vi "MH_WritePTURecordArr.vi"(0 "refnum":refnum<file>, 2 "TTTR Records":u32[](array[numeric]), 3 "error in":errorcluster) -> (6 "refnum en sortie":refnum<file>, 10 "error out":errorcluster)   [LabVIEW 2019]
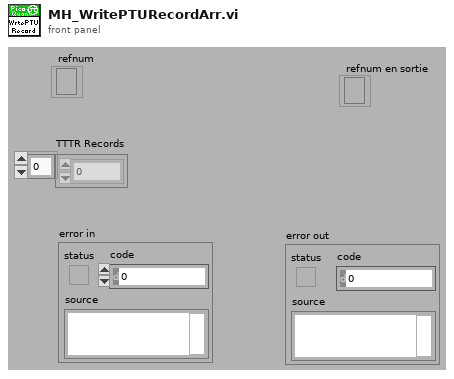
[diagram p1: front panel]
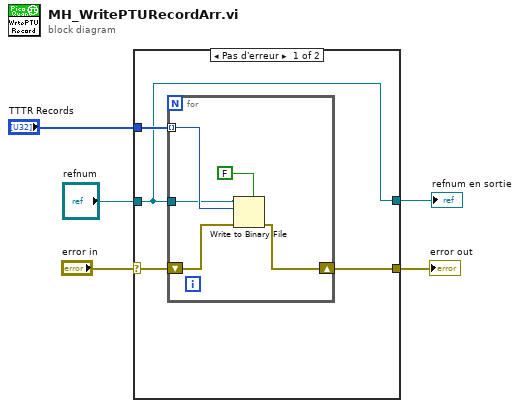
[diagram p0: block diagram]
diagram:
  n1 = case shown="Pas d'erreur" "error in" {
    selector: "error in" -> [w8 w16]
    tunnel: "refnum" -> [w6 w15]
    tunnel: [w9 w16] -> w4
    tunnel: "TTTR Records" -> [w7 _]
    tunnel: [w6 w15] -> w1
    frame No Error {
      n2 = for {
        tunnel: w6 -> [w12]
        shift-right: [w10] -> w9
        shift-left: w8 -> [w11]
        tunnel: w7 -> [w13] mode=indexing
        n3 = Write to Binary File(file (use dialog)=w12, data=w13, error in=w11, 5:FALSE ("ajouter une taille de tableau ou de chaîne ? (V)")) -> (error out=w10:errorcluster)  [unwired: 2 in, 2 out]
      }
    }
    frame Error {
    }
  }
  "error out" <- w4
  "refnum en sortie" <- w1
